vi "Load Subset.vi"(7 "Read channels":string[](array[string]), 8 "error in":errorcluster, 9 "Length":i32, 10 "Start Index":i32=-1, 11 "File Path":path=path "C:/Data/October_2025/102525/m003_111527_102525.tdms") -> (0 "error out":errorcluster={"status"=TRUE, "code"=-2532, "source"="TDMS Read in loacate subset.vi"}, 3 "file path out":path=path "\\\\myhome\\NHMFL/Projects/Pressure/Code/Alex/m006_092123.tdms", 5 "Data out":dbl[][](array[numeric]))   [LabVIEW 2024]
panel:
  out "Read channels out":string[](array[string])
  out "Waveform Graph 2":dbl[](graph)
  out "Waveform Graph":waveform(dbl)[](graph)
  in  "group name in":string="p"
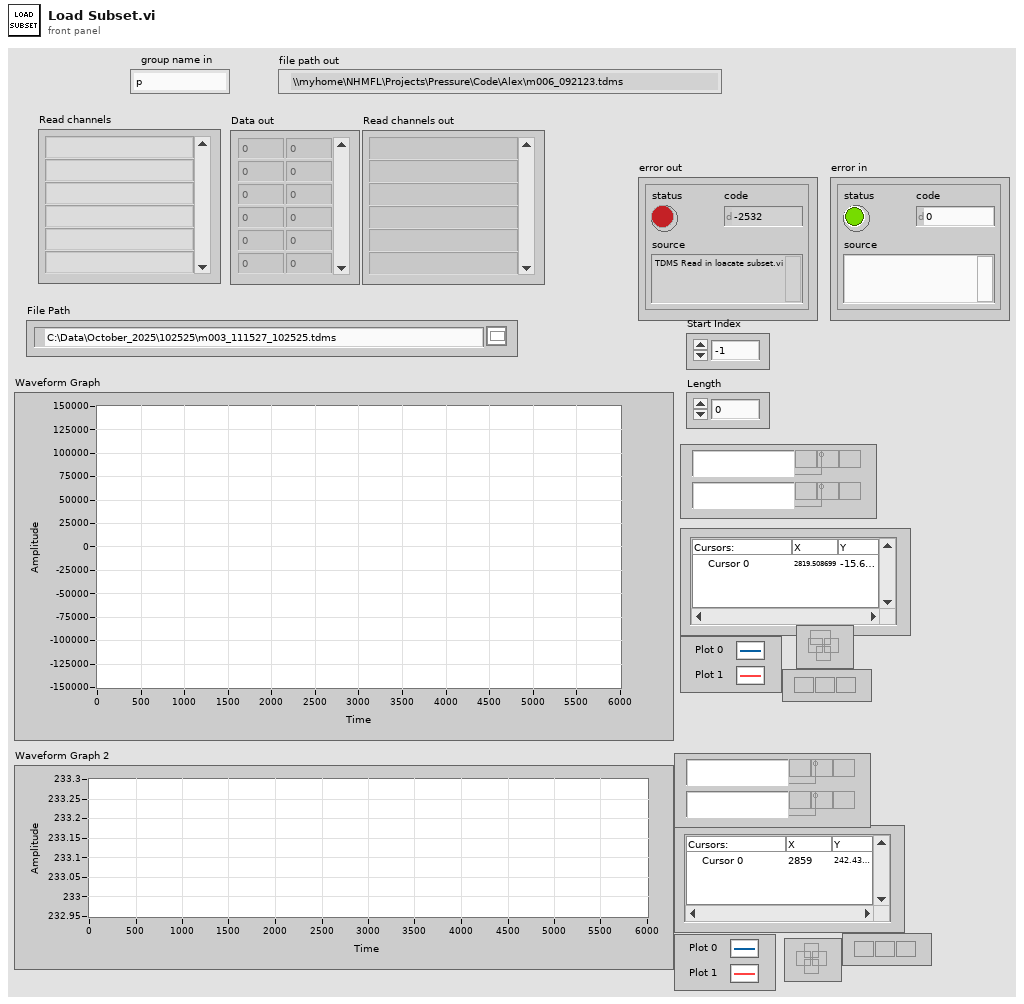
[diagram p1: front panel]
types:
  T1 = enum16{"open", "open or create", "create or replace", "create", "open (read-only)"}
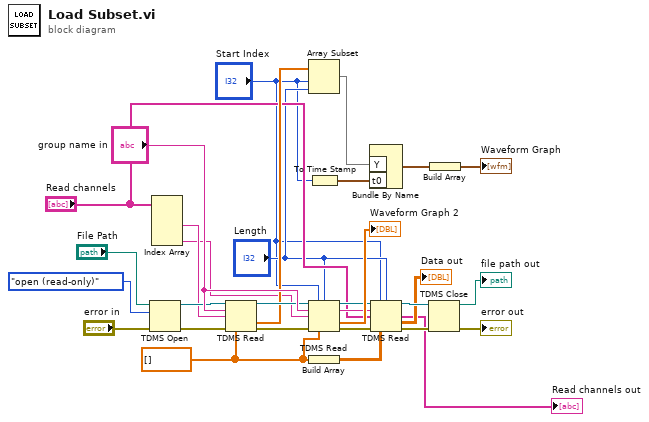
[diagram p0: block diagram]
diagram:
  w9 = dbl[] []
  n1 = TDMS Open(8:"error in", 10:T1."open (read-only)" ("operation (0:open)"), 11:"File Path") -> (0:w29:errorcluster, 3:w18:refnum<k34>)  [unwired: 4 in]
  n2 = Index Array(array="Read channels") -> (element #2=w5:string, element #4=w4:string)  [unwired: 4 in, 2 out]
  n3 = TDMS Read(0:w18, 5:"group name in", 7:w5, 11:w29, 12:w9) -> (4:w17:refnum<k34>, 10:w15:dbl[], 15:w16:errorcluster)  [unwired: 3 in, 3 out]
  n4 = Array Subset(array=w15, index="Start Index", length="Length") -> (w21:dbl[])
  n5 = TDMS Read(0:w17, 1:"Start Index", 2:"Length", 5:"group name in", 7:w4, 11:w16, 12:w9) -> (4:w11:refnum<k34>, 6:w12:string, 10:→"Waveform Graph 2":dbl[], 15:w14:errorcluster)  [unwired: 1 in, 2 out]
  n6 = Build Array(w9) -> (w8:dbl[][])
  n7 = To Time Stamp(1:"Start Index") -> (0:w19:timestamp)
  n8 = Bundle By Name("Y"=w21, "t0"=w19) -> (w27:waveform(dbl))  [unwired: 1 in]
  n9 = TDMS Read(0:w11, 1:"Start Index", 2:"Length", 5:w12, 7:"Read channels", 11:w14, 12:w8) -> (4:w10:refnum<k34>, 8:→"Read channels out":string[], 10:→"Data out":dbl[][], 15:w13:errorcluster)  [unwired: 1 in, 2 out]
  n10 = TDMS Close(8:w13, 11:w10) -> (0:→"error out":errorcluster, 3:→"file path out":path)
  n11 = Build Array(w27) -> (→"Waveform Graph":waveform(dbl)[])
